vi "run python script.vi"() -> ()   [LabVIEW 2020]
uses:
  Program Files (x86)/National Instruments/LabVIEW 2020/examples/Connectivity/Python/support/PythonVersionsEnum.ctl
panel:
  in  "stop":bool
  in  "Run Python":bool
  in  "function name":string
  in  "module path":path
  out "error out":errorcluster
  in  "error in (no error)":errorcluster
  in  "python version":T1
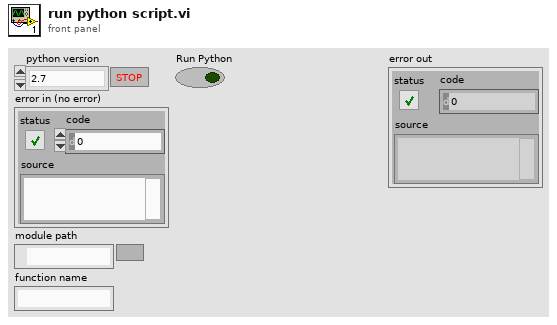
[diagram p1: front panel]
types:
  T1 = typedef "PythonVersionsEnum.ctl" = enum16{"2.7", "3.6"}
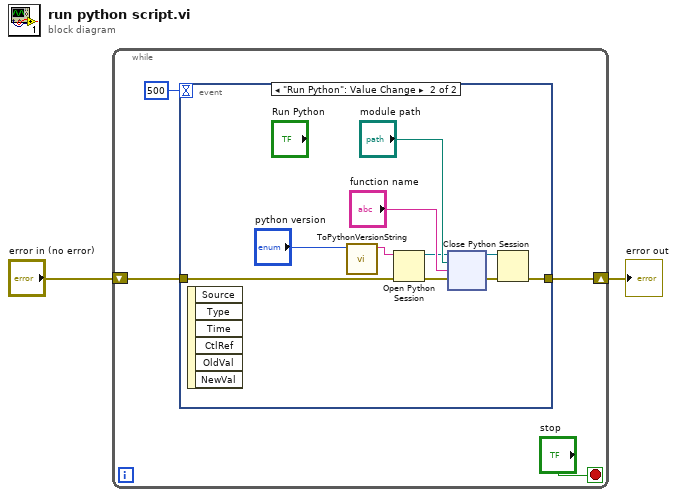
[diagram p0: block diagram]
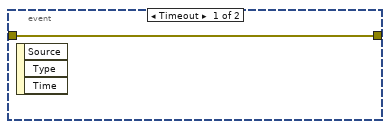
[diagram p2: hidden frame]
diagram:
  n1 = while {
    shift-right: [w3] -> w1
    shift-left: "error in (no error)" -> [w4]
    stop <- "stop" stop-if-true
    n2 = event shown="[1] \"Run Python\": Value Change" {
      selector: _ -> [_ _]
      dyn-events: _ -> [_ _]
      timeout: 500 -> [_ _]
      tunnel: w4 -> [w7 w9]
      tunnel: [w7 w8] -> w3
      event Timeout {
        n3 = event-data() -> ()  [unwired: 1 in, 3 out]
      }
      event "Run Python": Value Change {
        n4 = event-data() -> ()  [unwired: 1 in, 6 out]
        n5 = call "ToPythonVersionString.vi"("python version"="python version") -> ("python version string"=w14:string)  [unwired: 10 in]
        n6 = Open Python Session(python version=w14, 3:w9) -> (session out=w10:refnum<k35>, error out=w12:errorcluster)  [unwired: 1 in]
        n7 = node(w10, "module path", "function name", w12) -> (w11:refnum<k35>, w13:errorcluster)  [unwired: 2 in, 2 out]
        n8 = Close Python Session(session in=w11, error in=w13) -> (11:w8:errorcluster)
      }
    }
  }
  "error out" <- w1
